vi "MainSimplePid.vi"() -> ()   [LabVIEW 2019]
uses:
  <vilib>/Analysis/Matrix/Datatypes/RealMatrix.ctl
  <vilib>/userDefined/High Color/IMAQdx.ctl
  <vilib>/Platform/TimedLoop/XDataNode/timing_clust.ctl
  <vilib>/Platform/TimedLoop/XDataNode/nitl_modes.ctl
  <vilib>/Platform/TimedLoop/XDataNode/wakeup.ctl
  <vilib>/myRIO/Instrument Drivers/Onboard IO/AO/typedefs/AO Reference.ctl
  <vilib>/myRIO/Common/Instrument Driver Framework/Utilities/typedefs/myRIO Generic Hardware Reference.ctl
  <vilib>/myRIO/Common/Instrument Driver Framework/Utilities/typedefs/Hardware Version Enum.ctl
  <vilib>/myRIO/Common/Instrument Driver Framework/Utilities/typedefs/myRIO v1.0 Reference.ctl
  <vilib>/myRIO/Common/Instrument Driver Framework/Utilities/typedefs/Generic FPGA Reference.ctl
  <vilib>/myRIO/Common/Instrument Driver Framework/myRIO v1.0/AO/typedefs/AO Channels List.ctl
  <vilib>/myRIO/Common/Instrument Driver Framework/myRIO v1.0/AO/typedefs/AO Channels Enum.ctl
  <vilib>/myRIO/Common/Instrument Driver Framework/Utilities/typedefs/Analog Scaling Constants List.ctl
  <vilib>/myRIO/Common/Instrument Driver Framework/Utilities/typedefs/Analog Scaling Constants.ctl
  <vilib>/userDefined/High Color/nirio_resource_hc.ctl
  <vilib>/myRIO/Common/Instrument Driver Framework/myRIO v1.0/Encoder/typedefs/Encoder Signal Mode.ctl
  <vilib>/myRIO/Instrument Drivers/Onboard IO/Encoder/typedefs/Encoder Reference.ctl
  <vilib>/myRIO/Common/Instrument Driver Framework/myRIO v1.0/Encoder/typedefs/Encoder Channels Enum.ctl
  <vilib>/myRIO/Common/Instrument Driver Framework/myRIO v1.0/Encoder/typedefs/Encoder Configuration v1.0.ctl
  <vilib>/myRIO/Common/Instrument Driver Framework/Utilities/vis/Is FPGA Ref Available.vi
  <vilib>/myRIO/Common/Instrument Driver Framework/myRIO v1.0/AO/vis/myRIO v1.1 Open AO.vi
  <vilib>/myRIO/Instrument Drivers/Onboard IO/AO/vis/Write.vi
  <vilib>/myRIO/Common/Instrument Driver Framework/myRIO v1.0/Encoder/vis/myRIO v1.1 Open Encoder.vi
  <vilib>/myRIO/Instrument Drivers/Onboard IO/Encoder/vis/Read.vi
  <vilib>/myRIO/Common/Instrument Driver Framework/Utilities/vis/Validate Channels.vi
  <vilib>/myRIO/Common/Instrument Driver Framework/myRIO v1.0/AO/vis/myRIO v1.0 Reserve AO.vi
  <vilib>/myRIO/Common/Instrument Driver Framework/myRIO v1.0/Encoder/vis/myRIO v1.0 Reserve Encoder.vi
  <vilib>/myRIO/Common/Instrument Driver Framework/myRIO v1.0/AO/vis/myRIO v1.0 Build MUX Configuration AO.vi
  <vilib>/myRIO/Common/Instrument Driver Framework/myRIO v1.0/Resource Manager/vis/myRIO v1.0 Reserve Channel List.vi
  <vilib>/myRIO/Common/Instrument Driver Framework/myRIO v1.0/Encoder/vis/myRIO v1.0 Build MUX Configuration Encoder.vi
  <vilib>/myRIO/Common/Instrument Driver Framework/myRIO v1.0/Resource Manager/vis/myRIO v1.0 Reserve Channel.vi
  <vilib>/myRIO/Common/Instrument Driver Framework/myRIO v1.0/Resource Manager/vis/myRIO v1.0 Unreserve Channel.vi
  <vilib>/myRIO/Common/Instrument Driver Framework/myRIO v1.0/Resource Manager/vis/myRIO v1.0 Create Configuration List.vi
  <vilib>/myRIO/Common/Instrument Driver Framework/myRIO v1.0/Resource Manager/vis/myRIO v1.0 Build Mutex Name.vi
  <vilib>/Utility/VariantDataType/GetNumericInfo.vi
  <vilib>/Utility/error.llb/Error Cluster From Error Code.vi
  <vilib>/myRIO/Common/Instrument Driver Framework/myRIO v1.0/myRIO v1.1 Open.vi
  <vilib>/myRIO/Common/Instrument Driver Framework/myRIO v1.0/AO/vis/myRIO v1.0 Get Scaling Constants AO.vi
  <vilib>/myRIO/Common/Instrument Driver Framework/Utilities/vis/IO Manager.vi
  <vilib>/myRIO/Common/Instrument Driver Framework/Utilities/vis/Configuration Manager.vi
  <vilib>/myRIO/Common/Instrument Driver Framework/myRIO v1.0/myRIO v1.0 Close.vi
  <vilib>/myRIO/Common/Instrument Driver Framework/myRIO v1.0/AO/vis/myRIO v1.0 Write AO.vi
  <vilib>/Utility/file.llb/Write Delimited Spreadsheet (DBL).vi
  <vilib>/myRIO/Common/Instrument Driver Framework/myRIO v1.0/Resource Manager/vis/myRIO v1.0 Configure IO.vi
  <vilib>/myRIO/Common/Instrument Driver Framework/myRIO v1.0/Encoder/vis/myRIO v1.0 Configure Encoder.vi
  <vilib>/myRIO/Common/Instrument Driver Framework/myRIO v1.0/Encoder/vis/myRIO v1.0 Read Encoder.vi
  <vilib>/platform/TimedLoop/XDataNode/XDataNode.xnode
  <vilib>/myRIO/Express VI/Onboard IO/AO/AO Express VI.xnode
  <vilib>/myRIO/Instrument Drivers/Onboard IO/AO/vis/myRIO AO Open.xnode
  <vilib>/myRIO/Express VI/Onboard IO/Encoder/Encoder Express VI.xnode
  <vilib>/myRIO/Instrument Drivers/Onboard IO/Encoder/vis/myRIO Encoder Open.xnode
  <vilib>/myRIO/Common/Instrument Driver Framework/myRIO v1.0/Encoder/typedefs/Encoder Count Direction Enum.ctl
  <vilib>/Platform/TimedLoop/XDataNode/XDNodeRunTimeDep.lvlib
  <vilib>/myRIO/Instrument Drivers/Onboard IO/AO/AO.lvlib
  <vilib>/vision/driver/NI_Vision_Acquisition_Software.lvlib
  <vilib>/myRIO/Instrument Drivers/Onboard IO/Encoder/Encoder.lvlib
  <vilib>/vision/NI_Vision_Development_Module.lvlib
  <vilib>/Analysis/Matrix/NI_Matrix.lvlib
panel:
  in  "record_name":string
  out "record":T1
  out "step_recorded":dbl
  in  "stop_recording":bool
  in  "start_recording":bool
  out "recording":bool
  out "record_t":dbl[](array[numeric])
  out "target_angle_y_a_target":dbl(knob) scale=-45.0..45.0
  out "target_angle_x_a_target":dbl(knob) scale=-45.0..45.0
  in  "p_ki":dbl=-1.0
  in  "p_kd":dbl=-2000.0
  in  "p_kp":dbl
  out "y_angle":dbl(knob) scale=-45.0..45.0
  out "x_angle":dbl(knob) scale=-45.0..45.0
  out "y_error":dbl
  out "x_error":dbl
  in  "y_target":dbl(slide) scale=-1.0..1.0
  in  "x_target":dbl(slide) scale=-1.0..1.0
  out "y":dbl
  out "x":dbl
  out "camera":T2(plugin-control)
  in  "threshold":cluster{"Lower value":sgl, "Upper value":sgl}={"Lower value"=189.0, "Upper value"=255.0} {"Upper value" format="%.2f"; "Lower value" format="%.2f"}
  out "threshold":T2(plugin-control)
  out "x-y":u32
  out "y_input":dbl
  out "y_angle_error":dbl
  out "x_angle_error":dbl
  in  "stop":bool
  out "x_input":dbl
  in  "reset":bool
  in  "dt":dbl=20.0
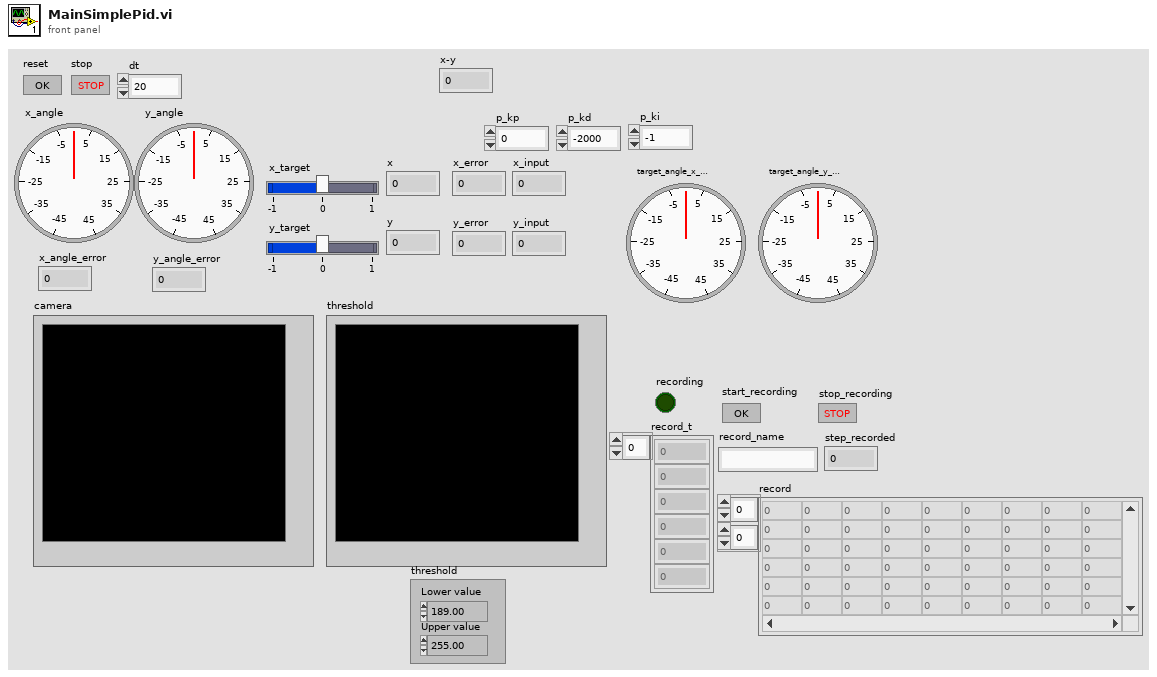
[diagram p1: front panel]
types:
  T1 = typedef "NI_Matrix.lvlib/RealMatrix.ctl" = dbl[][]
  T2 = typedef "IMAQ Image.ctl" = refnum<image>
  T3 = typedef "IMAQdx.ctl" = refnum<k21>
  T4 = typedef "XDNodeRunTimeDep.lvlib/timing_clust.ctl" = cluster{"Expected End [f-1]":u64, "Actual End [f-1]":u64, "Finished Late? [f-1]":bool, "Expected End [i-1]":u64, "Actual End [i-1]":u64, "Finished Late? [i-1]":bool, "Expected Start [i]":u64, "Actual Start [i]":u64, "Expected Start [f]":u64, "Actual Start [f]":u64, "Source Name":string, "Structure Name":string, "Period":i64, "Deadline":i64, "Offset":i64, "Start":i64, "Priority":i32, "Timeout":i32, "Mode":T5, "Wakeup Reason":T6, "Error":errorcluster, "Source Type":string, "Secondary Source Type":string, "Global End Time":u64, "Global Start Time":u64, "Frame Duration":u64, "Iteration Duration":u64, "Assigned CPU":i32, "I/O Scan Engine Mode":u32}
  T5 = typedef "XDNodeRunTimeDep.lvlib/nitl_modes.ctl" = enum32{"No Change", "Process missed periods, maintain original phase", "Discard missed periods, maintain original phase", "Process missed periods, ignore original phase", "Discard missed periods, ignore original phase"}
  T6 = typedef "XDNodeRunTimeDep.lvlib/wakeup.ctl" = enum32{"Normal", "Aborted", "Asynchronous wakeup", "Timing source error", "Timed loop error", "Timeout"}
  T7 = typedef "Encoder.lvlib/Encoder Reference.ctl" = cluster{"myRIO Reference":T8, "Encoder Channels Enum":T12}
  T8 = typedef "myRIO Generic Hardware Reference.ctl" = cluster{"myRIO Model":T9, "myRIO Hardware Reference":T10}
  T9 = typedef "Hardware Version Enum.ctl" = enum16{"Unknown", "myRIO-1900", "myRIO-1950", "roboRIO", "NI ELVIS RIO CM", "ELVIS III"}
  T10 = typedef "myRIO v1.0 Reference.ctl" = cluster{"Generic FPGA Reference":T11, "Allow multiple opens":bool}
  T11 = typedef "Generic FPGA Reference.ctl" = refnum<k20>
  T12 = typedef "Encoder Channels Enum.ctl" = enum16{"Not Connected", "C/ENC0", "C/ENC1", "A/ENC", "A/ENC0", "A/ENC1", "A/ENC2", "A/ENC3", "A/ENC4", "A/ENC5", "A/ENC6", "A/ENC7", "A/ENC8", "A/ENC9", "B/ENC", "B/ENC0", "B/ENC1", "B/ENC2", "B/ENC3", "B/ENC4", "B/ENC5", "B/ENC6", "B/ENC7", "B/ENC8", "B/ENC9", "DIO/ENC0", "DIO/ENC1", "DIO/ENC2", "DIO/ENC3", "DIO/ENC4"}
  T13 = typedef "Encoder Signal Mode.ctl" = enum16{"Quadrature phase signal", "Step and direction signal"}
  T14 = typedef "nirio_resource_hc.ctl" = tag
  T15 = typedef "AO.lvlib/AO Reference.ctl" = cluster{"myRIO Reference":T8, "AO Channel List":T16, "AO Scaling Constant List":T18}
  T16 = typedef "AO Channels List.ctl" = T17[]
  T17 = typedef "AO Channels Enum.ctl" = enum16{"Not Connected", "AudioOut/Left", "AudioOut/Right", "C/AO0", "C/AO1", "A/AO0", "A/AO1", "B/AO0", "B/AO1"}
  T18 = typedef "Analog Scaling Constants List.ctl" = T19[]
  T19 = typedef "Analog Scaling Constants.ctl" = cluster{"LSB Weight (Volts)":dbl, "Offset (Volts)":dbl, "Signed?":bool}
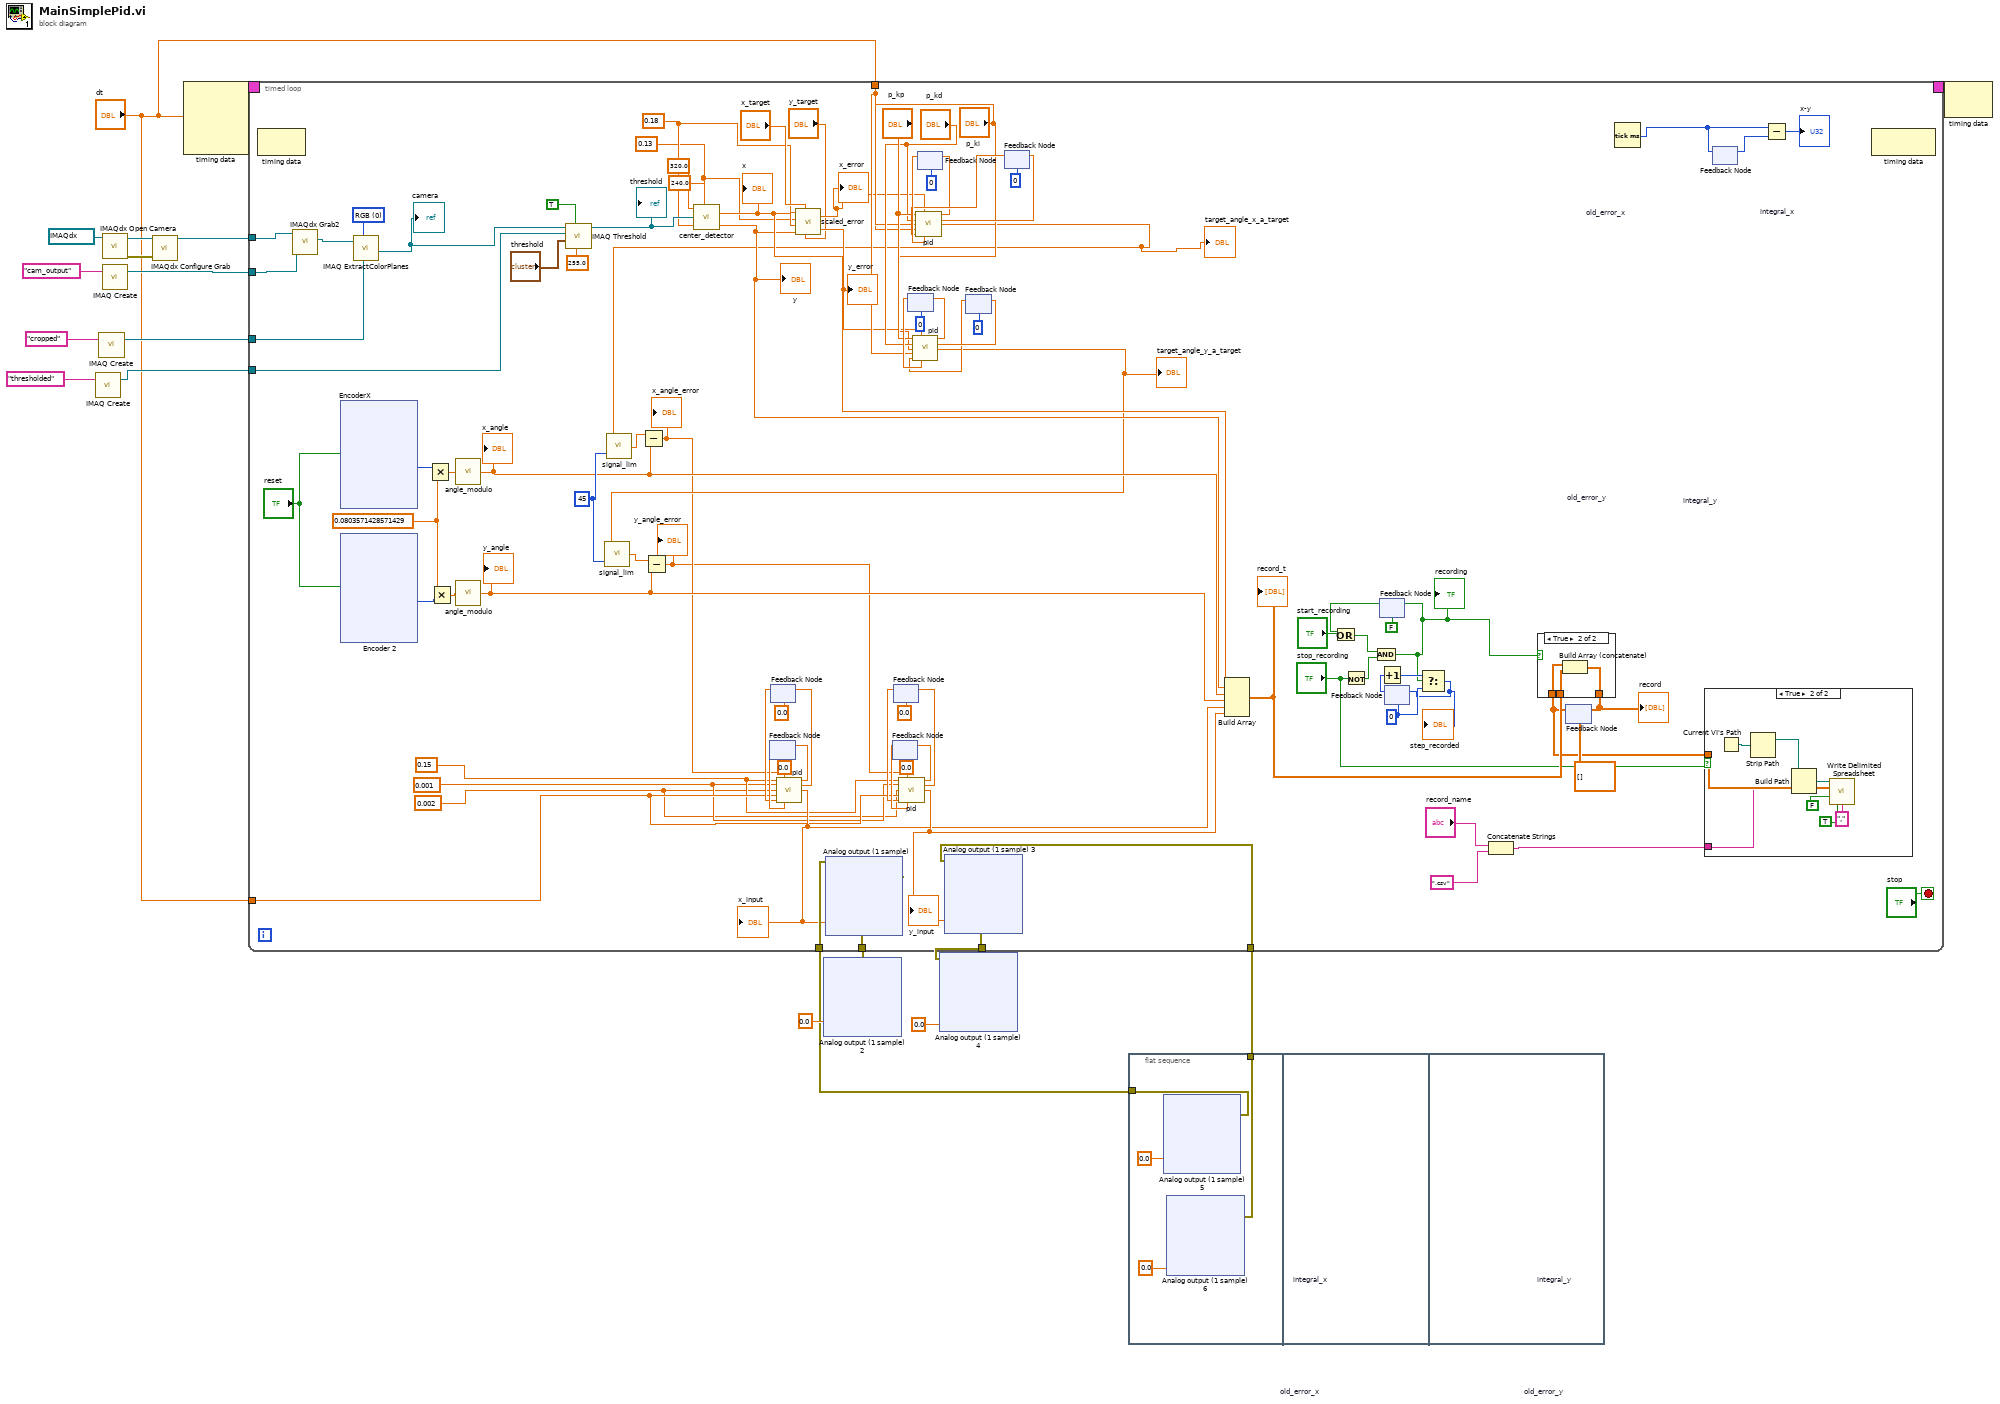
[diagram p0: block diagram]
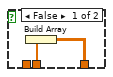
[diagram p3: hidden frame]
diagram:
  n1 = call "IMAQ Create"("Image Name"="thresholded") -> ("New Image"=w2:T2)  [unwired: 4 in, 1 out]
  n2 = call "IMAQ Create"("Image Name"="cropped") -> ("New Image"=w4:T2)  [unwired: 4 in, 1 out]
  n3 = call <vilib>:"IMAQdx Open Camera.vi"("Session In"=T3 "cam2") -> ("error out"=w11:errorcluster, "Session Out"=w12:T3)  [unwired: 9 in]
  n4 = call "IMAQ Create"("Image Name"="cam_output") -> ("New Image"=w13:T2)  [unwired: 4 in, 1 out]
  n5 = call <vilib>:"IMAQdx Configure Grab.vi"("error in"=w11, "Session In"=w12) -> ("Session Out"=w14:T3)  [unwired: 8 in, 1 out]
  n6 = node-c288("dt") -> (w19:T4)  [unwired: 3 in]
  n7 = timed-loop {
    timing: w19 -> [_]
    timing-out: [_] -> w18
    tunnel: w14 -> [w115]
    tunnel: w13 -> [w114]
    tunnel: "dt" -> [w23]
    tunnel: [w103] -> w9
    tunnel: [w99] -> w8
    tunnel: w7 -> [w98]
    tunnel: w6 -> [w97]
    tunnel: w4 -> [w53]
    tunnel: w2 -> [w57]
    tunnel: "dt" -> [w78]
    stop <- "stop" stop-if-true
    w20 = 0.002 ("ki")
    w21 = 0.001 ("kd")
    w22 = 0.15 ("kp")
    w42 = 0.13 ("m_y")
    w43 = 0.18 ("m_x")
    w56 = u16 0 items=["RGB", "HSL", "HSV", "HSI"] ("Color Mode")
    w68 = 0
    w104 = 45
    w112 = 0.0803571428571429
    n8 = node-c288() -> ()  [unwired: 1 in, 1 out]
    n9 = call <vilib>:"IMAQdx Grab2.vi"("Image In"=w114, "Session In"=w115) -> ("Image Out"=w55:T2)  [unwired: 6 in, 3 out]
    n10 = xnode "EncoderX"("Reset Counter"="reset") -> ("Counter Value"=w113:i32)  [unwired: 1 in, 3 out]
    n11 = xnode "Encoder 2"("Reset Counter"="reset") -> ("Counter Value"=w111:i32)  [unwired: 1 in, 3 out]
    n12 = call "IMAQ ExtractColorPlanes"("Blue or Luma or Val or Inten Plane"=w53, "Color Mode"=w56, "Image Src"=w55) -> ("Blue or Luma or Val or Inten Plane out"=w54:T2)  [unwired: 5 in, 3 out]
    "camera" <- w54
    n13 = Multiply(x=w113, y=w112) -> (x*y=w108:dbl)
    n14 = Multiply(x=w112, y=w111) -> (x*y=w107:dbl)
    n15 = call "angle_modulo.vi"("alpha"=w108) -> ("alpha_prime"=w77:dbl)
    "x_angle" <- w77
    n16 = call "angle_modulo.vi"("alpha"=w107) -> ("alpha_prime"=w76:dbl)
    "y_angle" <- w76
    n17 = call "IMAQ Threshold"("Replace Value"=sgl 255.0, "Keep/Replace Value (Replace)"=TRUE, "Range"="threshold", "Image Dst"=w57, "Image Src"=w54) -> ("Image Dst Out"=w50:T2)  [unwired: 5 in, 1 out]
    "threshold" <- w50
    n18 = call "center_detector.vi"("px_x"=320.0, "px_y"=240.0, "Image"=w50, "m_x"=w43, "m_y"=w42) -> ("x"=w45:dbl, "y"=w44:dbl)
    "x" <- w45
    "y" <- w44
    n19 = feedback #1 "old_error_x"(0.0 ("curr_err")) -> (w32:dbl)
    n20 = feedback #2 "integral_x"(0.0 ("curr_integral")) -> (w29:dbl)
    n21 = call "scaled_error.vi"("y_target"="y_target", "x_target"="x_target", "y"=w44, "x"=w45, "m_y"=w42, "m_x"=w43) -> ("err_y"=w49:dbl, "err_x"=w48:dbl)
    "x_error" <- w48
    "y_error" <- w49
    n22 = feedback #3 "old_error_y"(0.0 ("curr_err")) -> (w38:dbl)
    n23 = feedback #4 "integral_y"(0.0 ("curr_integral")) -> (w35:dbl)
    n24 = feedback #5 "old_error_y"(0) -> (w84:dbl)
    n25 = feedback #6 "old_error_x"(0) -> (w89:dbl)
    n26 = feedback #7 "integral_y"(0) -> (w82:dbl)
    n27 = call "pid.vi"("kp"="p_kp", "err"=w49, "kd"="p_kd", "ki"="p_ki", "dt"=w78, "intergral"=w82, "old_err"=w84) -> ("curr_err"=w85:dbl, "curr_integral"=w83:dbl, "y"=w41:dbl)  [unwired: 6 in]
    "target_angle_y_a_target" <- w41
    n28 = call "signal_lim.vi"("lim"=w104, "x"=w41) -> ("y"=w105:dbl)
    n29 = Subtract(x=w105, y=w76) -> (x-y=w24:dbl)
    "y_angle_error" <- w24
    n30 = call "pid.vi"("kp"=w22, "err"=w24, "kd"=w21, "ki"=w20, "dt"=w23, "intergral"=w35, "old_err"=w38) -> ("curr_err"=w39:dbl, "curr_integral"=w36:dbl, "y"=w27:dbl)  [unwired: 6 in]
    "y_input" <- w27
    n31 = feedback-in #3(w39) -> ()
    n32 = feedback-in #4(w36) -> ()
    n33 = feedback-in #5(w85) -> ()
    n34 = xnode "Analog output (1 sample) 3"("C/AO1 (AO1)"=w27, "error in (no error)"=w97) -> ("error out"=w99:errorcluster)
    n35 = feedback-in #7(w83) -> ()
    n36 = feedback #8 "integral_x"(0) -> (w87:dbl)
    n37 = call "pid.vi"("kp"="p_kp", "err"=w48, "kd"="p_kd", "ki"="p_ki", "dt"=w78, "intergral"=w87, "old_err"=w89) -> ("curr_err"=w86:dbl, "curr_integral"=w88:dbl, "y"=w40:dbl)  [unwired: 6 in]
    "target_angle_x_a_target" <- w40
    n38 = call "signal_lim.vi"("lim"=w104, "x"=w40) -> ("y"=w106:dbl)
    n39 = Subtract(x=w106, y=w77) -> (x-y=w25:dbl)
    "x_angle_error" <- w25
    n40 = call "pid.vi"("kp"=w22, "err"=w25, "kd"=w21, "ki"=w20, "dt"=w23, "intergral"=w29, "old_err"=w32) -> ("curr_err"=w33:dbl, "curr_integral"=w30:dbl, "y"=w26:dbl)  [unwired: 6 in]
    "x_input" <- w26
    n41 = feedback-in #1(w33) -> ()
    n42 = feedback-in #2(w30) -> ()
    n43 = xnode "Analog output (1 sample)"("C/AO0 (AO0)"=w26, "error in (no error)"=w98) -> ("error out"=w103:errorcluster)
    n44 = feedback-in #6(w86) -> ()
    n45 = feedback-in #8(w88) -> ()
    n46 = Build Array(w45, w44, w77, w76, w26, w27) -> (w65:dbl[])
    "record_t" <- w65
    n47 = Not(x="stop_recording") -> (.not. x?=w72:bool)
    n48 = feedback #9(FALSE) -> (w74:bool)
    n49 = Or(x=w74, y="start_recording") -> (x .or. y?=w73:bool)
    n50 = And(x=w73, y=w72) -> (x .and. y?=w66:bool)
    "recording" <- w66
    n51 = feedback-in #9(w66) -> ()
    n52 = feedback #10(w68) -> (w70:i32)
    n53 = Increment(x=w70) -> (x+1=w69:i32)
    n54 = Select(t=w69, s=w66, f=w68) -> (s? t:f=w67:i32)
    "step_recorded" <- w67
    n55 = feedback-in #10(w67) -> ()
    n56 = Concatenate Strings("record_name", ".csv") -> (w58:string)
    n57 = feedback #11(T1 [] ("Real Matrix")) -> (w61:T1)
    n58 = case shown="True" w66 {
      tunnel: w61 -> [_ w128]
      tunnel: [w124 w127] -> w63
      tunnel: w65 -> [w125 w126]
      frame False {
        n59 = Build Array(w125) -> (w124:T1)
      }
      frame True {
        n60 = Build Array (concatenate)(w128, w126) -> (w127:T1)
      }
    }
    "record" <- w63
    n61 = feedback-in #11(w63) -> ()
    n62 = Tick Count (ms)() -> (millisecond timer value=w102:u32)
    n63 = case shown="True" "stop_recording" {
      tunnel: w61 -> [_ w123]
      tunnel: w58 -> [_ w121]
      frame False {
      }
      frame True {
        n64 = Current VI's Path() -> (path=w119:path)
        n65 = Strip Path(path=w119) -> (stripped path=w118:path)  [unwired: 1 out]
        n66 = Build Path(base path=w118, name or relative path=w121) -> (appended path=w120:path)
        n67 = call-poly <vilib>:"Write Delimited Spreadsheet.vi"("file path (dialog if empty)"=w120, "2D data"=w123, "append to file? (new file:F)"=FALSE, "transpose? (no:F)"=TRUE, "delimiter (\\t)"="," ("delimiter (\\t)")) -> ()  [unwired: 9 in, 2 out]
      }
    }
    n68 = feedback-in #12(w102) -> ()
    n69 = feedback #12() -> (w101:u32)  [unwired: 1 in]
    n70 = Subtract(x=w102, y=w101) -> (x-y=→"x-y":u32)
    n71 = node-c288() -> ()  [unwired: 1 in, 1 out]
  }
  n72 = xnode "Analog output (1 sample) 2"("C/AO0 (AO0)"=0.0, "error in (no error)"=w9) -> ()  [unwired: 1 out]
  n73 = xnode "Analog output (1 sample) 4"("C/AO1 (AO1)"=0.0, "error in (no error)"=w8) -> ()  [unwired: 1 out]
  n74 = flat-sequence {
    tunnel: [w298] -> w7
    tunnel: [w297] -> w6
    frame #0 {
      n75 = xnode "Analog output (1 sample) 5"("C/AO0 (AO0)"=0.0) -> ("error out"=w298:errorcluster)  [unwired: 1 in]
      n76 = xnode "Analog output (1 sample) 6"("C/AO1 (AO1)"=0.0) -> ("error out"=w297:errorcluster)  [unwired: 1 in]
    }
    frame #1 {
    }
    frame #2 {
    }
  }
  n77 = node-c288(w18) -> ()  [unwired: 1 out]
